vi "Do.vi"(8 "error in (no error)":errorcluster, 10 "Actor in":refnum<class "Actor.lvclass">, 11 "Conceret Initialize Hot And Cold Source Unit Msg in":refnum<class "Conceret Initialize Hot And Cold Source Unit Msg.lvclass">) -> (0 "error out":errorcluster, 2 "Actor out":refnum<class "Actor.lvclass">)   [LabVIEW 2013, in "Hot And Cold Source Unit View.lvlib" / "Conceret Initialize Hot And Cold Source Unit Msg.lvclass"]
doc: "(<B>Filename</B>: Actor Framework.lvlib:Message.lvclass:Do.vi)\n\nDefines what a message does when it is received by an actor. Generally, a message instructs an actor to invoke one of its methods.\n\nBy default, this method does nothing. A child class must override it to define behavior. Create a child class by using the Actor Framework Message Maker dialog box."
uses:
  Conceret Initialize Hot And Cold Source Unit Msg.lvclass
  <vilib>/ActorFramework/Actor/Actor.lvclass
  Hot And Cold Source Unit View/Hot And Cold Source Unit View.lvclass
  Models/Hot And Cold Source Unit Model Messages/Abstract Initialize Hot And Cold Source Unit Msg/Abstract Initialize Hot And Cold Source Unit Msg.lvclass
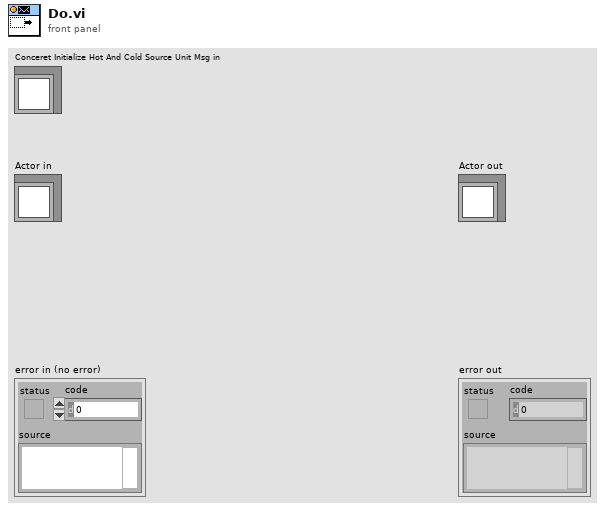
[diagram p1: front panel]
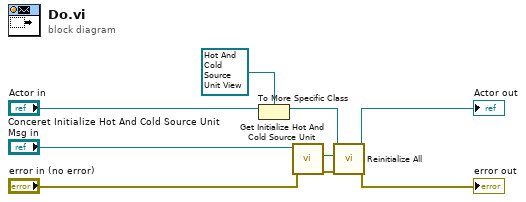
[diagram p0: block diagram]
diagram:
  n1 = To More Specific Class(target class=refnum<class "Hot And Cold Source Unit View.lvclass"> refnum ("Hot And Cold Source Unit View.lvlib:Hot And Cold Source Unit View.lvclass"), reference="Actor in") -> (specific class reference=w6:refnum<class "Hot And Cold Source Unit View.lvclass">)  [unwired: 1 in, 1 out]
  n2 = call "Get Initialize Hot And Cold Source Unit.vi"("error in (no error)"="error in (no error)", "Abstract Initialize Hot And Cold Source Unit Msg in"="Conceret Initialize Hot And Cold Source Unit Msg in") -> ("error out"=w5:errorcluster, "Initialize Hot And Cold Source Unit"=w1:bool)  [unwired: 7 in, 1 out]
  n3 = call "Reinitialize All.vi"("error in (no error)"=w5, "Initialize Hot And Cold Source Unit"=w1, "Hot And Cold Source Unit View in"=w6) -> ("error out"=→"error out":errorcluster, "Hot And Cold Source Unit View out"=→"Actor out":refnum<class "Hot And Cold Source Unit View.lvclass">)  [unwired: 7 in]
